vi "testError.vi"() -> ()   [LabVIEW 2019, in "AssertionTest.lvlib" / "AssertStringNotContainsStringIgnoringCase.lvlib"]
uses:
  AssertStringNotContainsStringIgnoringCase.lvlib
  <vilib>/Utility/error.llb/Error Cluster From Error Code.vi
  <vilib>/ErrorRing/Error Ring.xnode
  Assertion/Assertion.lvlib
panel:
  out "error out":errorcluster
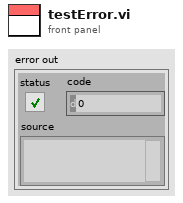
[diagram p1: front panel]
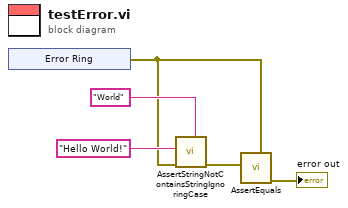
[diagram p0: block diagram]
diagram:
  n1 = xnode "Error Ring"() -> ("error out"=w2:errorcluster)
  n2 = call "AssertStringNotContainsStringIgnoringCase.vi"("Needle"="World", "error in (no error)"=w2, "Haystack"="Hello World!") -> ("error out"=w3:errorcluster)  [unwired: 8 in]
  n3 = call "AssertEquals.vi"("Expected"=w2, "Actual"=w3) -> ("error out"=→"error out":errorcluster)  [unwired: 9 in]
